vi "img test10(occlusion attempt 1).vi"() -> ()   [LabVIEW 2013]
uses:
  <vilib>/vision/NI_Vision_Development_Module.lvlib
panel:
  out "Image 4":T1(plugin-control)
  in  "frame jump":i32=3
  in  "speed":u32(slide)=200
  in  "start":i32(slide) step=219843704 scale=0.0..124012.0
  out "Image 3":T1(plugin-control)
  out "Image 2":T1(plugin-control)
  in  "AVI Path":path=path "C:/Users/Kokum Weeratunga/Desktop/img processing/ChongWei vs LinDan (japan open 2010).avi"
  # "thilini hendahewa"
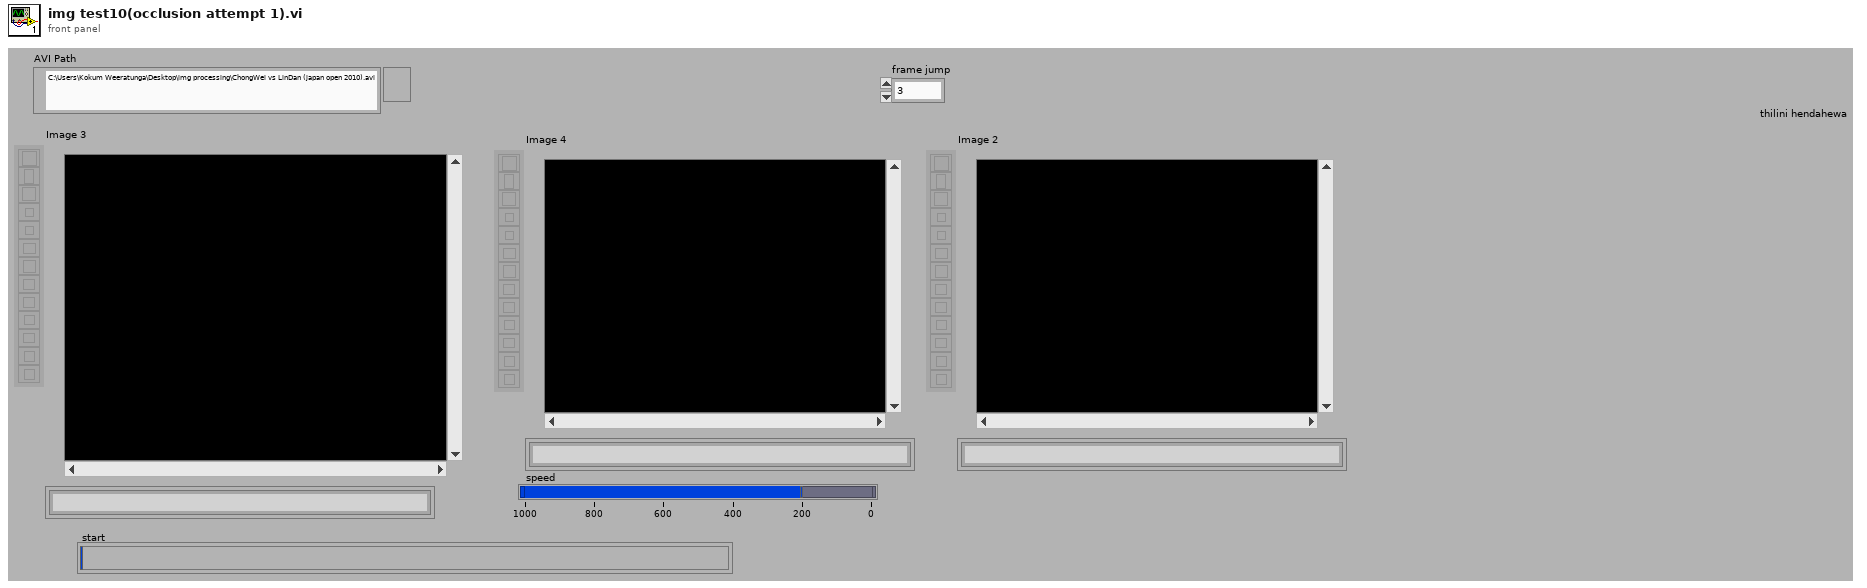
[diagram p1: front panel]
types:
  T1 = typedef "IMAQ Image.ctl" = refnum<image>
  T2 = typedef "Image Type" = u32
  T3 = typedef "AviRefnum.ctl" = refnum<k1>
  T4 = typedef "Particle Parameters" = i32
  T5 = cluster{"Numeric":dbl, "Numeric":dbl, "Numeric":dbl, "Numeric":dbl}
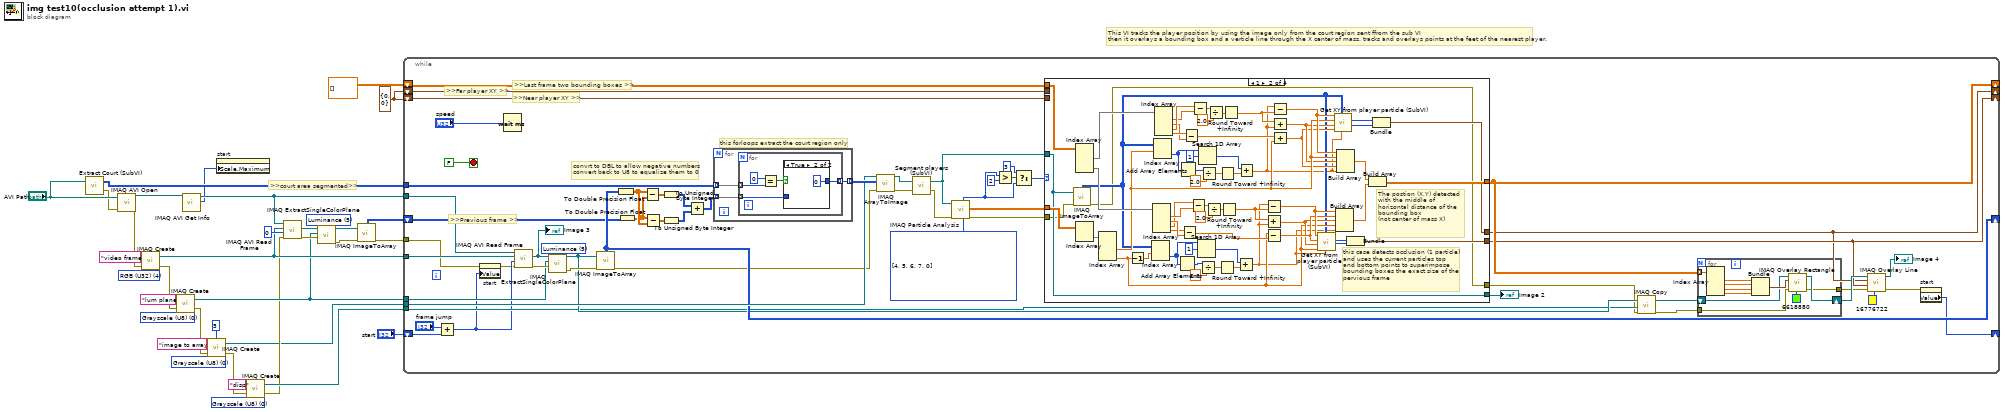
[diagram p0: block diagram]
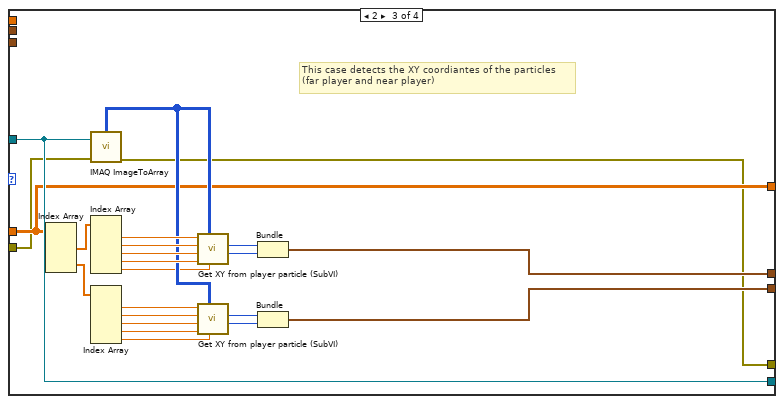
[diagram p3: hidden frame]
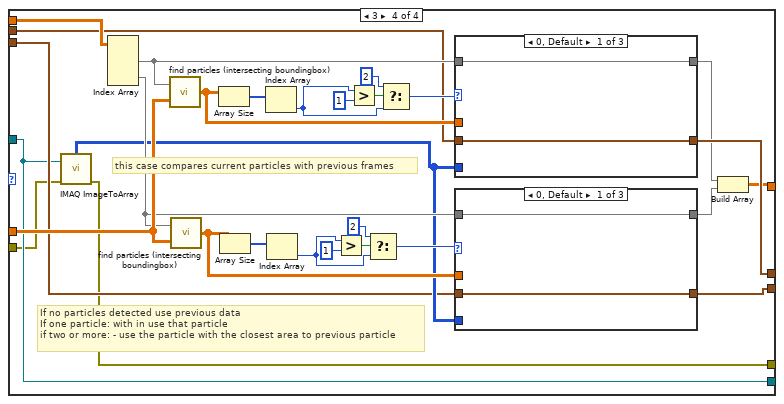
[diagram p4: hidden frame]
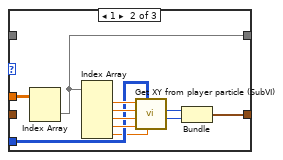
[diagram p5: hidden frame]
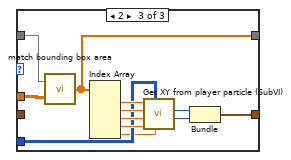
[diagram p6: hidden frame]
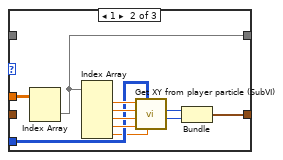
[diagram p7: hidden frame]
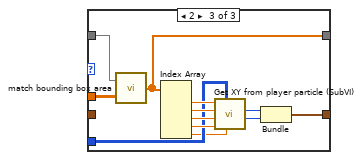
[diagram p8: hidden frame]
diagram:
  w6 = cluster{"X coordinate":i32, "Y coordinate":i32} {"X coordinate"=0, "Y coordinate"=0}
  w19 = T2 0 items=["Grayscale (U8)", "Grayscale (I16)", "Grayscale (SGL)", "Complex (CSG)", "RGB (U32)", "HSL (U32)", "RGB (U64)", "Grayscale (U16)"] ("Image Type")
  w26 = 5 items=["Red", "Green", "Blue", "Hue", "Saturation", "Luminance", "Value", "Intensity"] ("Color Plane")
  w28 = T2 0 items=["Grayscale (U8)", "Grayscale (I16)", "Grayscale (SGL)", "Complex (CSG)", "RGB (U32)", "HSL (U32)", "RGB (U64)", "Grayscale (U16)"] ("Image Type")
  w32 = T2 0 items=["Grayscale (U8)", "Grayscale (I16)", "Grayscale (SGL)", "Complex (CSG)", "RGB (U32)", "HSL (U32)", "RGB (U64)", "Grayscale (U16)"] ("Image Type")
  w30 = T2 4 items=["Grayscale (U8)", "Grayscale (I16)", "Grayscale (SGL)", "Complex (CSG)", "RGB (U32)", "HSL (U32)", "RGB (U64)", "Grayscale (U16)"] ("Image Type")
  # ">>court area segmented>>"
  # "This VI tracks the player position by using the image only from the court region sent ffrom the sub VI\nthen it overlays a bounding box and a verticle line through the X center of mass. tracks and overlays points at the feet of the nearest player."
  n1 = call "Extract Court (SubVI).vi"("AVI Path"="AVI Path") -> ("error out"=w34:errorcluster, "Court pixels out"=w9:u8[][])  [unwired: 1 in]
  n2 = call "IMAQ AVI Open"("error in (no error)"=w34, "AVI Path"="AVI Path") -> ("error out"=w15:errorcluster, "Avi Refnum"=w4:T3)  [unwired: 8 in]
  n3 = call "IMAQ Create"("Image Name"="video frame", "Image Type"=w30, "error in (no error)"=w15) -> ("New Image"=w23:T1, "error out"=w14:errorcluster)  [unwired: 2 in]
  n4 = call "IMAQ Create"("Image Name"="lum plane", "Image Type"=w32, "error in (no error)"=w14) -> ("New Image"=w22:T1, "error out"=w13:errorcluster)  [unwired: 2 in]
  n5 = call "IMAQ AVI Get Info"("Avi Refnum"=w4) -> ("Number of Frames"=w2:u32, "Avi Refnum (duplicate)"=w3:T3)  [unwired: 6 in, 3 out]
  n6 = call "IMAQ Create"("Border Size"=5, "Image Name"="image to array", "Image Type"=w28, "error in (no error)"=w13) -> ("New Image"=w8:T1, "error out"=w12:errorcluster)  [unwired: 1 in]
  n7 = property on="start" class="Slide (strict)"("Scale.Maximum"=w2) -> ()  [unwired: 2 in, 2 out]
  n8 = call "IMAQ Create"("Image Name"="disp", "Image Type"=w19, "error in (no error)"=w12) -> ("New Image"=w17:T1, "error out"=w11:errorcluster)  [unwired: 2 in]
  n9 = call "IMAQ AVI Read Frame"("error in (no error)"=w11, "Frame Number"=u32 0, "Image"=w23, "Avi Refnum"=w3) -> ("error out"=w25:errorcluster, "Image Out"=w27:T1)  [unwired: 4 in, 2 out]
  n10 = call "IMAQ ExtractSingleColorPlane"("Color Plane"=w26, "error in (no error)"=w25, "Image Dst"=w22, "Image Src"=w27) -> ("error out"=w16:errorcluster, "Image Dst Out"=w20:T1)  [unwired: 6 in]
  n11 = call "IMAQ ImageToArray"("error in (no error)"=w16, "Image"=w20) -> ("error out"=w1:errorcluster, "Image Pixels (U8)"=w21:u8[][])  [unwired: 2 in, 3 out]
  n12 = while {
    tunnel: w3 -> [w45]
    tunnel: w23 -> [w73]
    tunnel: w9 -> [w90]
    tunnel: w22 -> [w74]
    tunnel: w8 -> [w87]
    shift-right: [w86] -> _
    shift-left: w21 -> [w85]
    tunnel: w17 -> [w52]
    shift-right: [w59] -> _
    shift-left: dbl[][] [] ("Particle Measurements (Pixels)") -> [w60]
    shift-right: [w36] -> _
    shift-left: w6 -> [w37]
    shift-right: [w39] -> _
    shift-left: w6 -> [w38]
    shift-right: [w40] -> _
    shift-left: "start" -> [w47]
    tunnel: w1 -> [w43]
    stop <- FALSE stop-if-true
    w75 = T4[] [4, 5, 6, 7, 0] items=["Center of Mass X", "Center of Mass Y", "First Pixel X", "First Pixel Y", "Bounding Rect Left", "Bounding Rect Top", "Bounding Rect Right", "Bounding Rect Bottom", "Max Feret Diameter Start X", "Max Feret Diameter Start Y", "Max Feret Diameter End X", "Max Feret Diameter End Y", "Max Horiz. Segment Length Left", "Max Horiz. Segment Length Right", "Max Horiz. Segment Length Row", "-", "Bounding Rect Width", "Bounding Rect Height", "Bounding Rect Diagonal", "Perimeter", "Convex Hull Perimeter", "Holes' Perimeter", "Max Feret Diameter", "Equivalent Ellipse Major Axis", "Equivalent Ellipse Minor Axis", "Equivalent Ellipse Minor Axis (Feret)", "Equivalent Rect Long Side", "Equivalent Rect Short Side", "Equivalent Rect Diagonal", "Equivalent Rect Short Side (Feret)", "Average Horiz. Segment Length", "Average Vert. Segment Length", "Hydraulic Radius", "Waddel Disk Diameter", "-", "Area", "Holes' Area", "Particle & Holes' Area", "Convex Hull Area", "Image Area", "-", "Number of Holes", "Number of Horiz. Segments", "Number of Vert. Segments", "-", "Orientation", "Max Feret Diameter Orientation", "-", "% Area/Image Area", "% Area/(Particle & Holes' Area)", "Ratio of Equivalent Ellipse Axes", "Ratio of Equivalent Rect Sides", "-", "Elongation Factor", "Compactness Factor", "Heywood Circularity Factor", "Type Factor", "-", "Sum X", "Sum Y", "Sum XX", "Sum XY", "Sum YY", "Sum XXX", "Sum XXY", "Sum XYY", "Sum YYY", "-", "Moment of Inertia XX", "Moment of Inertia XY", "Moment of Inertia YY", "Moment of Inertia XXX", "Moment of Inertia XXY", "Moment of Inertia XYY", "Moment of Inertia YYY", "Norm. Moment of Inertia XX", "Norm. Moment of Inertia XY", "Norm. Moment of Inertia YY", "Norm. Moment of Inertia XXX", "Norm. Moment of Inertia XXY", "Norm. Moment of Inertia XYY", "Norm. Moment of Inertia YYY", "Hu Moment 1", "Hu Moment 2", "Hu Moment 3", "Hu Moment 4", "Hu Moment 5", "Hu Moment 6", "Hu Moment 7"] ("Pixel Measurements")
    w91 = 5 items=["Red", "Green", "Blue", "Hue", "Saturation", "Luminance", "Value", "Intensity"] ("Color Plane")
    # ">>Last frame two bounding boxes >>"
    # ">>Far player XY >>"
    # ">>Near player XY >>"
    # ">>Previous frame >>"
    # "convrt to DBL to allow negative numbers\nconvert back to U8 to equalize them to 0"
    # "this forloops extract the court region only"
    n13 = Add(x="frame jump", y=w47) -> (x+y=w44:i32)
    n14 = property on="start" class="Slide (strict)"(error in=w43, "Value"=w44) -> (error out=w42:errorcluster)  [unwired: 1 in, 1 out]
    n15 = Wait (ms)(milliseconds to wait="speed") -> ()  [unwired: 1 out]
    n16 = call "IMAQ AVI Read Frame"("error in (no error)"=w42, "Frame Number"=w44, "Image"=w73, "Avi Refnum"=w45) -> ("error out"=w92:errorcluster, "Image Out"=w70:T1)  [unwired: 4 in, 2 out]
    "Image 3" <- w70
    n17 = call "IMAQ ExtractSingleColorPlane"("Color Plane"=w91, "error in (no error)"=w92, "Image Dst"=w74, "Image Src"=w70) -> ("error out"=w77:errorcluster, "Image Dst Out"=w53:T1)  [unwired: 6 in]
    n18 = call "IMAQ ImageToArray"("error in (no error)"=w77, "Image"=w53) -> ("error out"=w76:errorcluster, "Image Pixels (U8)"=w86:u8[][])  [unwired: 2 in, 3 out]
    n19 = To Double Precision Float(number=w86) -> (double precision float=w81:dbl[][])
    n20 = To Double Precision Float(number=w85) -> (double precision float=w80:dbl[][])
    n21 = Subtract(x=w81, y=w80) -> (x-y=w79:dbl[][])
    n22 = Subtract(x=w80, y=w81) -> (x-y=w78:dbl[][])
    n23 = To Unsigned Byte Integer(number=w79) -> (unsigned 8bit integer=w84:u8[][])
    n24 = To Unsigned Byte Integer(number=w78) -> (unsigned 8bit integer=w83:u8[][])
    n25 = Add(x=w84, y=w83) -> (x+y=w82:u8[][])
    n26 = for {
      tunnel: w90 -> [w274] mode=indexing
      tunnel: [w273] -> w88 mode=indexing
      tunnel: w82 -> [w272] mode=indexing
      n27 = for {
        tunnel: w274 -> [w279] mode=indexing
        tunnel: [w276] -> w273 mode=indexing
        tunnel: w272 -> [w275] mode=indexing
        n28 = Equal?(x=u8 0, y=w279) -> (x = y?=w277:bool)
        n29 = case shown="True" w277 {
          tunnel: [w280 u8 0 ("x")] -> w276
          tunnel: w275 -> [w280 _]
          frame False {
          }
          frame True {
          }
        }
      }
    }
    n30 = call "IMAQ ArrayToImage"("error in (no error)"=w76, "Image Pixels (U8)"=w88, "Image"=w87) -> ("error out"=w71:errorcluster, "Image Out"=w72:T1)  [unwired: 7 in]
    n31 = call "Segment players (SubVI).vi"("error In"=w71, "Image In"=w72) -> ("error out"=w64:errorcluster, "Image Out"=w62:T1)
    n32 = call "IMAQ Particle Analysis"("error in (no error)"=w64, "Pixel Measurements"=w75, "Image"=w62) -> ("error out"=w63:errorcluster, "Particle Measurements (Pixels)"=w61:dbl[][], "Number of Particles"=w66:i32)  [unwired: 3 in, 3 out]
    n33 = Greater?(x=w66, y=2) -> (0:w69:bool)
    n34 = Select(t=3 ("y"), s=w69, f=w66) -> (s? t:f=w65:i32)
    n35 = case shown="1" w65 {
      tunnel: [w107 w134 w188 w198] -> w57
      tunnel: w61 -> [_ w169 w174 w218]
      tunnel: w63 -> [w104 w110 w171 w194]
      tunnel: w62 -> [w107 w134 w188 w198]
      tunnel: [w105 w118 w176 w200] -> w39
      tunnel: [w106 w125 w175 w199] -> w36
      tunnel: [w108 w135 w174 w195] -> w59
      tunnel: w60 -> [w108 w159 _ w221]
      tunnel: w37 -> [w106 _ _ w206]
      tunnel: w38 -> [w105 _ _ w201]
      tunnel: [w104 w109 w170 w193] -> w50
      frame 0, Default {
        # "This case identifies frames where no particles are detected and keeps the same values from the\nprevious frame"
      }
      frame 1 {
        # "The postion (X,Y) detected with the middle of \nhorizontal distance of the bounding box\n(not center of mass X)"
        # "this case detects occlusion (1 particle)\nand uses the current particles top \nand bottom points to superimpose \nbounding boxes the exact size of the \npervious frame"
        n36 = call "IMAQ ImageToArray"("error in (no error)"=w110, "Image"=w134) -> ("error out"=w109:errorcluster, "Image Pixels (U8)"=w117:u8[][])  [unwired: 2 in, 3 out]
        n37 = Index Array(array=w159) -> (element #1=w167:dbl[], element #2=w139:dbl[])  [unwired: 4 in]
        n38 = Index Array(array=w169) -> (element=w168:dbl[])  [unwired: 2 in]
        n39 = Index Array(array=w168) -> (element #2=w130:dbl, element #4=w121:dbl)  [unwired: 4 in, 2 out]
        n40 = Decrement(x=w121) -> (x-1=w132:dbl)
        n41 = Index Array(array=w117, index (row)=w132) -> (element=w154:u8[])  [unwired: 1 in]
        n42 = Index Array(array=w139) -> (element #1=w143:dbl, element #2=w146:dbl, element #3=w142:dbl, element #4=w145:dbl)  [unwired: 4 in]
        n43 = Index Array(array=w117, index (row)=w130) -> (element=w147:u8[])  [unwired: 1 in]
        n44 = Index Array(array=w167) -> (element #1=w163:dbl, element #2=w160:dbl, element #3=w164:dbl, element #4=w161:dbl)  [unwired: 4 in]
        n45 = Add Array Elements(numeric array=w154) -> (sum=w155:u8)
        n46 = Add Array Elements(numeric array=w147) -> (sum=w151:u8)
        n47 = Subtract(x=w145, y=w146) -> (x-y=w133:dbl)
        n48 = Subtract(x=w161, y=w160) -> (x-y=w138:dbl)
        n49 = Subtract(x=w142, y=w143) -> (x-y=w141:dbl)
        n50 = Subtract(x=w164, y=w163) -> (x-y=w165:dbl)
        n51 = Search 1D Array(1D array=w154, element=u8 1) -> (index of element=w153:i32)  [unwired: 1 in]
        n52 = Search 1D Array(1D array=w147, element=u8 1) -> (index of element=w152:i32)  [unwired: 1 in]
        n53 = Divide(x=w155, y=2.0) -> (x/y=w156:dbl)
        n54 = Divide(x=w151, y=2.0) -> (x/y=w150:dbl)
        n55 = Divide(x=w141, y=2.0) -> (x/y=w144:dbl)
        n56 = Divide(x=w165, y=2.0) -> (x/y=w162:dbl)
        n57 = Round Toward +Infinity(x=w156) -> (ceil(x): smallest int >= x=w115:dbl)
        n58 = Round Toward +Infinity(x=w150) -> (ceil(x): smallest int >= x=w114:dbl)
        n59 = Round Toward +Infinity(x=w144) -> (ceil(x): smallest int >= x=w116:dbl)
        n60 = Round Toward +Infinity(x=w162) -> (ceil(x): smallest int >= x=w113:dbl)
        n61 = Add(x=w153, y=w115) -> (x+y=w111:dbl)
        n62 = Add(x=w152, y=w114) -> (x+y=w112:dbl)
        n63 = Subtract(x=w111, y=w116) -> (x-y=w124:dbl)
        n64 = Add(x=w116, y=w111) -> (x+y=w122:dbl)
        n65 = Subtract(x=w121, y=w133) -> (x-y=w123:dbl)
        n66 = Subtract(x=w112, y=w113) -> (x-y=w131:dbl)
        n67 = Add(x=w113, y=w112) -> (x+y=w129:dbl)
        n68 = Add(x=w138, y=w130) -> (x+y=w128:dbl)
        n69 = call "Get XY from player particle (SubVI).vi"("Center of mass X"=w111, "Image in Pixels (U8)"=w117, "Particle bounding rect bottom"=w121, "Particle bounding rect right"=w122, "Particle bounding rect top"=w123, "Particle bounding rect left"=w124) -> ("Y coordinate"=w119:i32, "X coordinate"=w120:i32)  [unwired: 2 in]
        n70 = call "Get XY from player particle (SubVI).vi"("Center of mass X"=w112, "Image in Pixels (U8)"=w117, "Particle bounding rect bottom"=w128, "Particle bounding rect right"=w129, "Particle bounding rect top"=w130, "Particle bounding rect left"=w131) -> ("Y coordinate"=w126:i32, "X coordinate"=w127:i32)  [unwired: 2 in]
        n71 = Build Array(w124, w123, w122, w121, w111) -> (w136:dbl[])
        n72 = Build Array(w131, w130, w129, w128, w112) -> (w137:dbl[])
        n73 = Bundle("X coordinate"=w120, "Y coordinate"=w119) -> (w118:cluster{"X coordinate":i32, "Y coordinate":i32})  [unwired: 1 in]
        n74 = Build Array(w137, w136) -> (w135:dbl[][])
        n75 = Bundle("X coordinate"=w127, "Y coordinate"=w126) -> (w125:cluster{"X coordinate":i32, "Y coordinate":i32})  [unwired: 1 in]
      }
      frame 2 {
        # "This case detects the XY coordiantes of the particles\n(far player and near player)"
        n76 = Index Array(array=w174) -> (element #1=w182:dbl[], element #2=w181:dbl[])  [unwired: 4 in]
        n77 = call "IMAQ ImageToArray"("error in (no error)"=w171, "Image"=w188) -> ("error out"=w170:errorcluster, "Image Pixels (U8)"=w183:u8[][])  [unwired: 2 in, 3 out]
        n78 = Index Array(array=w182) -> (element #1=w192:dbl, element #2=w191:dbl, element #3=w190:dbl, element #4=w189:dbl, element #5=w173:dbl)  [unwired: 5 in]
        n79 = Index Array(array=w181) -> (element #1=w184:dbl, element #2=w185:dbl, element #3=w186:dbl, element #4=w187:dbl, element #5=w172:dbl)  [unwired: 5 in]
        n80 = call "Get XY from player particle (SubVI).vi"("Center of mass X"=w173, "Image in Pixels (U8)"=w183, "Particle bounding rect bottom"=w189, "Particle bounding rect right"=w190, "Particle bounding rect top"=w191, "Particle bounding rect left"=w192) -> ("Y coordinate"=w179:i32, "X coordinate"=w180:i32)  [unwired: 2 in]
        n81 = call "Get XY from player particle (SubVI).vi"("Center of mass X"=w172, "Image in Pixels (U8)"=w183, "Particle bounding rect bottom"=w187, "Particle bounding rect right"=w186, "Particle bounding rect top"=w185, "Particle bounding rect left"=w184) -> ("Y coordinate"=w177:i32, "X coordinate"=w178:i32)  [unwired: 2 in]
        n82 = Bundle("X coordinate"=w180, "Y coordinate"=w179) -> (w175:cluster{"X coordinate":i32, "Y coordinate":i32})  [unwired: 1 in]
        n83 = Bundle("X coordinate"=w178, "Y coordinate"=w177) -> (w176:cluster{"X coordinate":i32, "Y coordinate":i32})  [unwired: 1 in]
      }
      frame 3 {
        # "If no particles detected use previous data\nIf one particle: with in use that particle\nif two or more: - use the particle with the closest area to previous particle"
        # "this case compares current particles with previous frames"
        n84 = call "IMAQ ImageToArray"("error in (no error)"=w194, "Image"=w198) -> ("error out"=w193:errorcluster, "Image Pixels (U8)"=w202:u8[][])  [unwired: 2 in, 3 out]
        n85 = Index Array(array=w221) -> (element #1=w217:dbl[], element #2=w205:dbl[])  [unwired: 4 in]
        n86 = call "find particles (intersecting boundingbox).vi"("Particle Measurements in (bounding boxes)"=w218, "bounding box in"=w217) -> ("Particles within bounding box"=w216:dbl[][])
        n87 = call "find particles (intersecting boundingbox).vi"("Particle Measurements in (bounding boxes)"=w218, "bounding box in"=w205) -> ("Particles within bounding box"=w203:dbl[][])
        n88 = Array Size(array=w216) -> (size(s)=w220:i32[])
        n89 = Array Size(array=w203) -> (size(s)=w219:i32[])
        n90 = Index Array(array=w220) -> (element=w208:i32)  [unwired: 1 in]
        n91 = Index Array(array=w219) -> (element=w209:i32)  [unwired: 1 in]
        n92 = Greater?(x=w209, y=1) -> (0:w212:bool)
        n93 = Greater?(x=w208, y=1) -> (0:w213:bool)
        n94 = Select(t=2 ("y"), s=w212, f=w209) -> (s? t:f=w204:i32)
        n95 = Select(t=2 ("y"), s=w213, f=w208) -> (s? t:f=w207:i32)
        n96 = case shown="0, Default" w207 {
          tunnel: w217 -> [w248 _ w263]
          tunnel: w216 -> [_ w259 w262]
          tunnel: [w248 w250 w261] -> w197
          tunnel: w202 -> [_ w252 w265]
          tunnel: [w247 w251 w264] -> w199
          tunnel: w206 -> [w247 _ _]
          frame 0, Default {
          }
          frame 1 {
            n97 = Index Array(array=w259) -> (element=w250:dbl[])  [unwired: 2 in]
            n98 = Index Array(array=w250) -> (element #1=w256:dbl, element #2=w255:dbl, element #3=w254:dbl, element #4=w253:dbl, element #5=w249:dbl)  [unwired: 5 in]
            n99 = call "Get XY from player particle (SubVI).vi"("Center of mass X"=w249, "Image in Pixels (U8)"=w252, "Particle bounding rect bottom"=w253, "Particle bounding rect right"=w254, "Particle bounding rect top"=w255, "Particle bounding rect left"=w256) -> ("Y coordinate"=w257:i32, "X coordinate"=w258:i32)  [unwired: 2 in]
            n100 = Bundle("X coordinate"=w258, "Y coordinate"=w257) -> (w251:cluster{"X coordinate":i32, "Y coordinate":i32})  [unwired: 1 in]
          }
          frame 2 {
            n101 = call "match bounding box area.vi"("particle measurements (bounding box)"=w262, "bounding box in"=w263) -> ("matching bounding box"=w261:dbl[])
            n102 = Index Array(array=w261) -> (element #1=w269:dbl, element #2=w268:dbl, element #3=w267:dbl, element #4=w266:dbl, element #5=w260:dbl)  [unwired: 5 in]
            n103 = call "Get XY from player particle (SubVI).vi"("Center of mass X"=w260, "Image in Pixels (U8)"=w265, "Particle bounding rect bottom"=w266, "Particle bounding rect right"=w267, "Particle bounding rect top"=w268, "Particle bounding rect left"=w269) -> ("Y coordinate"=w270:i32, "X coordinate"=w271:i32)  [unwired: 2 in]
            n104 = Bundle("X coordinate"=w271, "Y coordinate"=w270) -> (w264:cluster{"X coordinate":i32, "Y coordinate":i32})  [unwired: 1 in]
          }
        }
        n105 = case shown="0, Default" w204 {
          tunnel: w205 -> [w223 _ w238]
          tunnel: w203 -> [_ w234 w237]
          tunnel: [w223 w225 w236] -> w196
          tunnel: w202 -> [_ w227 w240]
          tunnel: [w222 w226 w239] -> w200
          tunnel: w201 -> [w222 _ _]
          frame 0, Default {
          }
          frame 1 {
            n106 = Index Array(array=w234) -> (element=w225:dbl[])  [unwired: 2 in]
            n107 = Index Array(array=w225) -> (element #1=w231:dbl, element #2=w230:dbl, element #3=w229:dbl, element #4=w228:dbl, element #5=w224:dbl)  [unwired: 5 in]
            n108 = call "Get XY from player particle (SubVI).vi"("Center of mass X"=w224, "Image in Pixels (U8)"=w227, "Particle bounding rect bottom"=w228, "Particle bounding rect right"=w229, "Particle bounding rect top"=w230, "Particle bounding rect left"=w231) -> ("Y coordinate"=w232:i32, "X coordinate"=w233:i32)  [unwired: 2 in]
            n109 = Bundle("X coordinate"=w233, "Y coordinate"=w232) -> (w226:cluster{"X coordinate":i32, "Y coordinate":i32})  [unwired: 1 in]
          }
          frame 2 {
            n110 = call "match bounding box area.vi"("particle measurements (bounding box)"=w237, "bounding box in"=w238) -> ("matching bounding box"=w236:dbl[])
            n111 = Index Array(array=w236) -> (element #1=w244:dbl, element #2=w243:dbl, element #3=w242:dbl, element #4=w241:dbl, element #5=w235:dbl)  [unwired: 5 in]
            n112 = call "Get XY from player particle (SubVI).vi"("Center of mass X"=w235, "Image in Pixels (U8)"=w240, "Particle bounding rect bottom"=w241, "Particle bounding rect right"=w242, "Particle bounding rect top"=w243, "Particle bounding rect left"=w244) -> ("Y coordinate"=w245:i32, "X coordinate"=w246:i32)  [unwired: 2 in]
            n113 = Bundle("X coordinate"=w246, "Y coordinate"=w245) -> (w239:cluster{"X coordinate":i32, "Y coordinate":i32})  [unwired: 1 in]
          }
        }
        n114 = Build Array(w197, w196) -> (w195:dbl[][])
      }
    }
    "Image 2" <- w57
    n115 = call "IMAQ Copy"("error in (no error)"=w50, "Image Dst"=w52, "Image Src"=w53) -> ("error out"=w49:errorcluster, "Image Dst Out"=w51:T1)  [unwired: 3 in]
    n116 = for {
      shift-right: [w95] -> w55
      shift-left: w51 -> [w99]
      tunnel: w59 -> [w97] mode=indexing
      tunnel: w49 -> [w94]
      tunnel: [w93] -> w48
      n117 = Index Array(array=w97) -> (element #1=w103:dbl, element #2=w102:dbl, element #3=w101:dbl, element #4=w96:dbl)  [unwired: 4 in]
      n118 = Bundle("Numeric"=w103, "Numeric"=w102, "Numeric"=w101, "Numeric"=w96) -> (w100:T5)  [unwired: 1 in]
      n119 = call "IMAQ Overlay Rectangle"("Color"=u32 6618880, "error in (no error)"=w94, "Rectangle"=w100, "Image"=w99) -> ("error out"=w93:errorcluster, "Image Out"=w95:T1)  [unwired: 6 in]
    }
    n120 = call "IMAQ Overlay Line"("Color"=u32 16776722, "error in (no error)"=w48, "End Point"=w39, "Start Point"=w36, "Image"=w55) -> ("error out"=w41:errorcluster, "Image Out"=→"Image 4":T1)  [unwired: 5 in]
    n121 = property on="start" class="Slide (strict)"(error in=w41) -> ("Value"=w40:i32)  [unwired: 1 in, 2 out]
  }
